vi "DECODIFICAR ESTADO LED.vi"(11 "COMANDO":string) -> (3 "concatenated string":string)   [LabVIEW 2019]
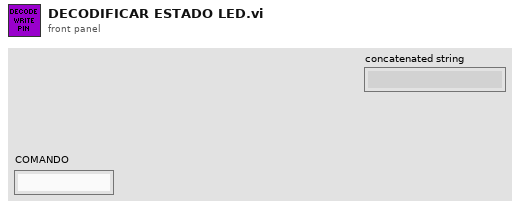
[diagram p1: front panel]
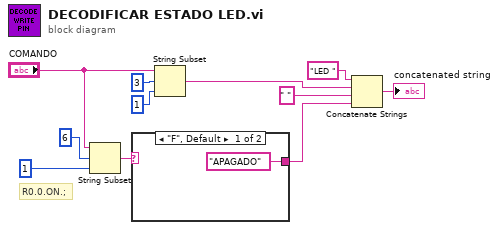
[diagram p0: block diagram]
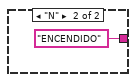
[diagram p2: hidden frame]
diagram:
  # "R0.0.ON.;"
  n1 = String Subset(string="COMANDO", offset (0)=6, length (rest)=1 ("length (rest)")) -> (substring=w6:string)
  n2 = case shown="\"F\", Default" w6 {
    tunnel: ["APAGADO" "ENCENDIDO"] -> w2
    frame "F", Default {
    }
    frame "N" {
    }
  }
  n3 = String Subset(string="COMANDO", offset (0)=3, length (rest)=1 ("length (rest)")) -> (substring=w4:string)
  n4 = Concatenate Strings("LED " ("string"), w4, " " ("string"), w2) -> (→"concatenated string":string)
